vi "Msg.vi"(7 "Actor in":refnum<class "Actor.lvclass">, 11 "Event Last Ack Msg in":refnum<class "Event Last Ack Msg.lvclass">) -> (5 "Actor out":refnum<class "Actor.lvclass">)   [LabVIEW 2021, in "jettl.lvlib" / "Event Last Ack.lvlib" / "Event Last Ack Msg.lvclass"]
uses:
  Event Last Ack Msg.lvclass
  jettl/Actor/Actor.lvclass
  Event Last Ack/Event Last Ack.lvclass
  Event Last Ack Msg.lvclass/Event Last Ack Msg.ctl
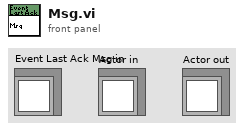
[diagram p1: front panel]
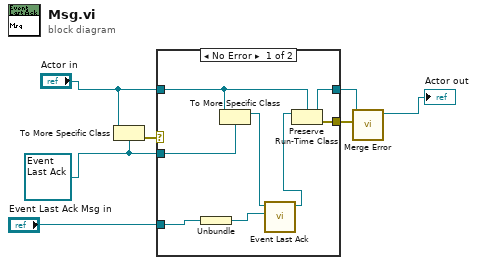
[diagram p0: block diagram]
diagram:
  w2 = refnum<class "Event Last Ack.lvclass"> refnum ("Event Last Ack.lvlib:Event Last Ack.lvclass")
  n1 = To More Specific Class(target class=w2, reference="Actor in") -> (error out=w7:errorcluster)  [unwired: 1 in, 1 out]
  n2 = case shown="No Error" w7 {
    selector: w7 -> [_ w16]
    tunnel: [w13 w17] -> w5
    tunnel: "Actor in" -> [w14 w17]
    tunnel: w2 -> [w15 _]
    tunnel: [w12 w16] -> w6
    tunnel: "Event Last Ack Msg in" -> [w9 _]
    frame No Error {
      n3 = Unbundle(w9) -> (w8:refnum<class "Event Actor.lvclass">)
      n4 = To More Specific Class(target class=w15, reference=w14) -> (specific class reference=w11:refnum<class "Event Last Ack.lvclass">)  [unwired: 1 in, 1 out]
      n5 = call-dynamic "Event Last Ack.vi"("Event Actor"=w8, "Event Last Ack in"=w11) -> ("Event Last Ack out"=w10:refnum<class "Event Last Ack.lvclass">)  [unwired: 9 in]
      n6 = Preserve Run-Time Class(object in=w10, 2:w14) -> (object out=w13:refnum<class "Actor.lvclass">, error out=w12:errorcluster)  [unwired: 1 in]
    }
    frame Error {
    }
  }
  n7 = call-dynamic "Merge Error.vi"("Error"=w6, "Set Error in"=w5) -> ("Set Error out"=→"Actor out":refnum<class "Actor.lvclass">)  [unwired: 9 in]
